vi "XY.vi"() -> ()   [LabVIEW 2011]
panel:
  out "Numeric 2":dbl
  out "Numeric":dbl
  out "Latched Cordinates":i32[](array[numeric])
  out "?":i32[](array[numeric])
  out "Original Image":T1(plugin-control)
  # "Cordniates"
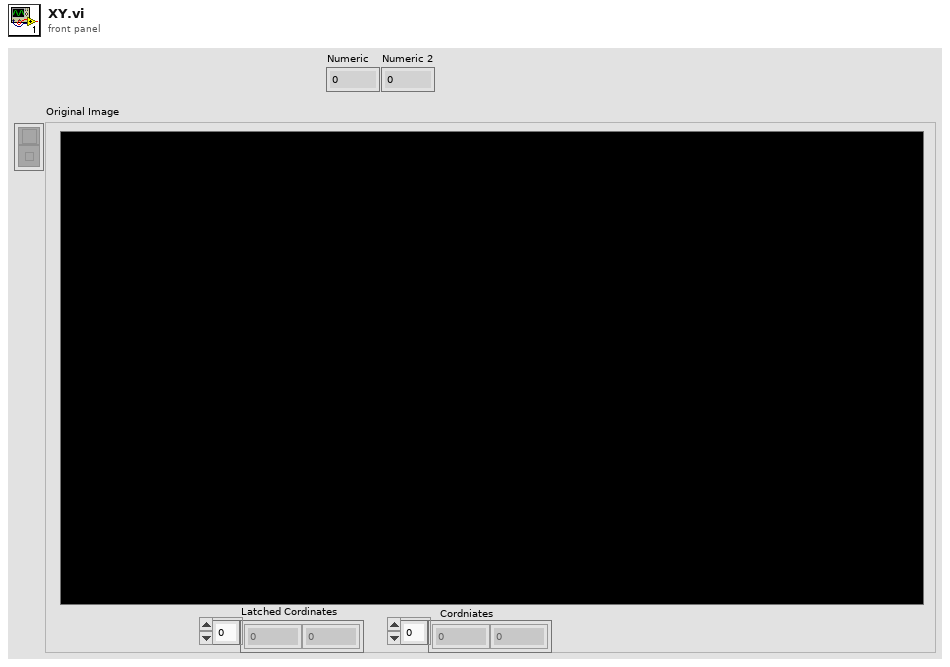
[diagram p1: front panel]
types:
  T1 = typedef "IMAQ Image.ctl" = refnum<image>
  T2 = typedef "Image Type" = u32
  T3 = cluster{"Coordinates[0]":i32, "Coordinates[1]":i32, "Coordinates[2]":i32, "Coordinates[3]":i32, "Coordinates[4]":i32, "Coordinates[5]":i32, "Coordinates[6]":i32, "Coordinates[7]":i32, "Coordinates[8]":i32}
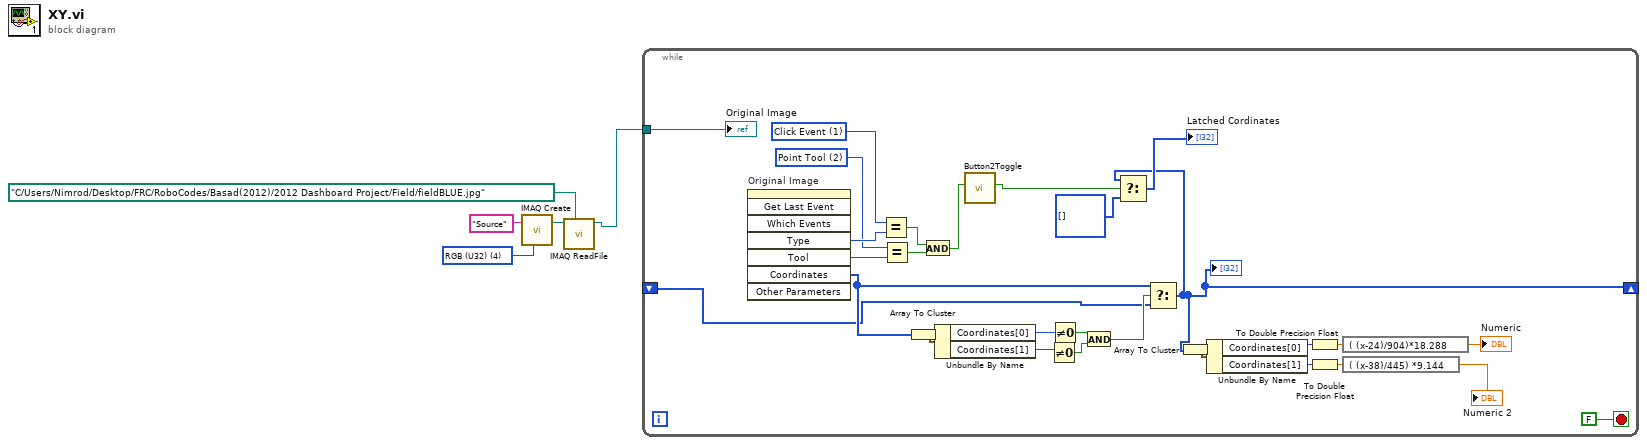
[diagram p0: block diagram]
diagram:
  w1 = T2 4 items=["Grayscale (U8)", "Grayscale (I16)", "Grayscale (SGL)", "Complex (CSG)", "RGB (U32)", "HSL (U32)", "RGB (U64)", "Grayscale (U16)"] ("Image Type")
  n1 = call "IMAQ Create"("Image Name"="Source", "Image Type"=w1) -> ("New Image"=w3:T1)  [unwired: 2 in, 2 out]
  n2 = call "IMAQ ReadFile"("File Path"=path "C:/Users/Nimrod/Desktop/FRC/RoboCodes/Basad(2012)/2012 Dashboard Project/Field/fieldBLUE.jpg", "Image"=w3) -> ("Image Out"=w2:T1)  [unwired: 5 in, 4 out]
  n3 = while {
    tunnel: w2 -> [w27]
    shift-right: [w12] -> _
    shift-left: _ -> [w17]
    stop <- FALSE stop-if-true
    w28 = 2 items=["None", "Selection Tool", "Point Tool", "Line Tool", "Rectangle Tool", "Oval Tool", "Polygon Tool", "ClosedFreehandTool", "Annulus Tool", "Rotated Rectangle Tool", "Zoom Tool", "Pan Tool", "Polyline Tool", "Freehand Tool"] ("Tool")
    w29 = 1 items=["No Event"=0, "Click Event"=1, "Draw Event"=2, "Size Event"=4, "Scroll Event"=5, "Double Click Event"=8] ("Type")
    n4 = invoke on="Original Image" class="ImageControl" method="Get Last Event"() -> ("Type"=w30:i32, "Tool"=w33:i32, "Coordinates"=w18:i32[])  [unwired: 8 in, 5 out]
    n5 = Equal?(x=w29, y=w30) -> (x = y?=w31:bool)
    n6 = Equal?(x=w28, y=w33) -> (x = y?=w32:bool)
    n7 = Array To Cluster(array=w18) -> (cluster=w24:T3)
    n8 = And(x=w31, y=w32) -> (x .and. y?=w25:bool)
    n9 = Unbundle By Name(w24) -> ("Coordinates[0]"=w22:i32, "Coordinates[1]"=w20:i32)
    n10 = call "Button2Toggle.vi"("Boolean"=w25) -> ("Latched Boolean"=w16:bool)  [unwired: 9 in, 1 out]
    n11 = Not Equal To 0?(x=w20) -> (x != 0?=w21:bool)
    n12 = Not Equal To 0?(x=w22) -> (x != 0?=w23:bool)
    n13 = And(x=w23, y=w21) -> (x .and. y?=w19:bool)
    n14 = Select(t=w18, s=w19, f=w17) -> (s? t:f=w12:i32[])
    "?" <- w12
    n15 = Select(t=w12, s=w16, f=i32[] [] ("Coordinates")) -> (s? t:f=→"Latched Cordinates":i32[])
    n16 = Array To Cluster(array=w12) -> (cluster=w13:T3)
    n17 = Unbundle By Name(w13) -> ("Coordinates[0]"=w11:i32, "Coordinates[1]"=w8:i32)
    n18 = To Double Precision Float(number=w11) -> (double precision float=w9:dbl)
    n19 = To Double Precision Float(number=w8) -> (double precision float=w10:dbl)
    n20 = expression code="( (x-24)/904)*18.288"(w9) -> (→"Numeric":dbl)
    n21 = expression code="( (x-38)/445) *9.144"(w10) -> (→"Numeric 2":dbl)
    "Original Image" <- w27
  }
